vi "copyScriptToTestDir.vi"(8 "error in (no error)":errorcluster, 10 "Path in":path, 11 "FileNeologist in":refnum<class "FileNeologist.lvclass">) -> (0 "error out":errorcluster, 2 "Path out":path, 3 "FileNeologist out":refnum<class "FileNeologist.lvclass">)   [LabVIEW 2011, in "Tools.lvlib" / "Filing.lvlib" / "FileNeologist.lvclass"]
uses:
  FileNeologist.lvclass
  FileNeologist.lvclass/FileNeologist.ctl
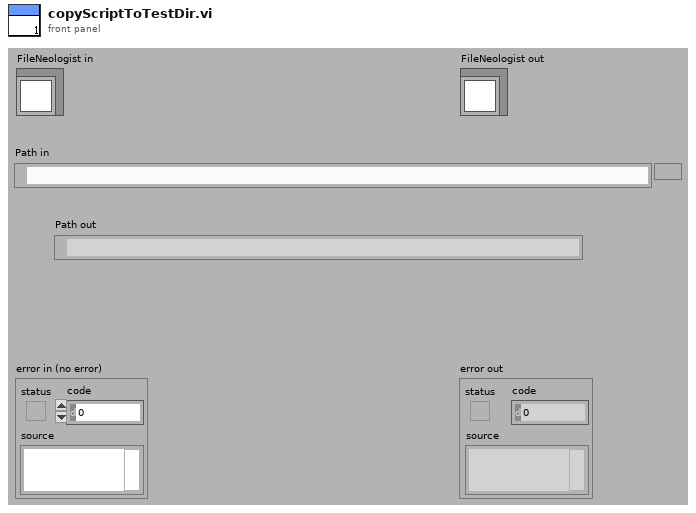
[diagram p1: front panel]
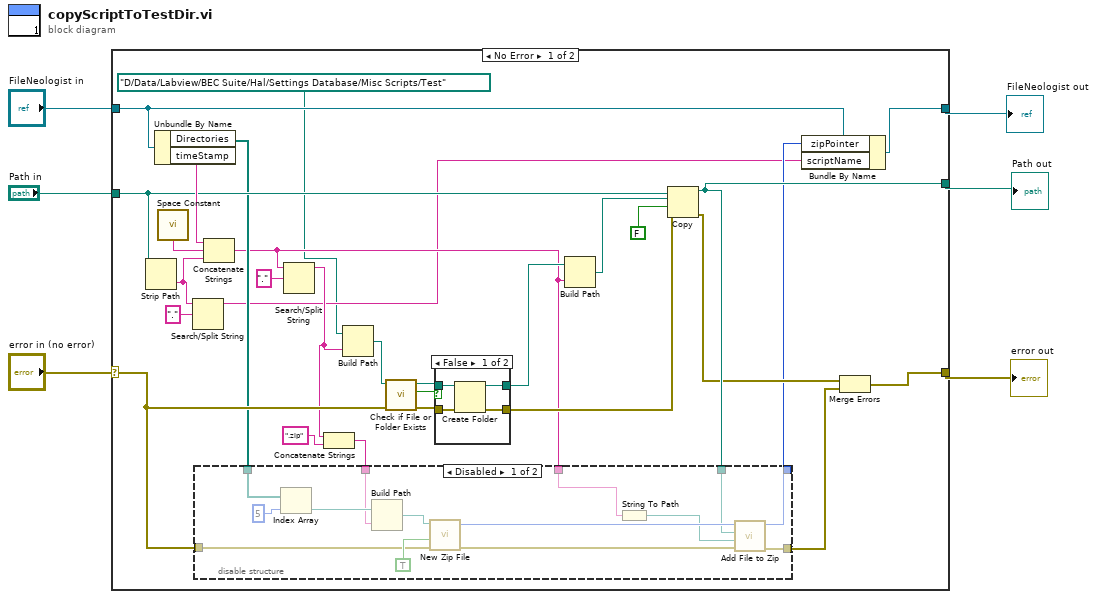
[diagram p0: block diagram]
diagram:
  n1 = case shown="No Error" "error in (no error)" {
    selector: "error in (no error)" -> [w23 w57]
    tunnel: [w20 w57] -> w5
    tunnel: [w11 w56] -> w3
    tunnel: "FileNeologist in" -> [w12 w56]
    tunnel: "Path in" -> [w25 _]
    tunnel: [w22 _] -> w1
    frame No Error {
      n2 = Strip Path(path=w25) -> (name=w9:string)  [unwired: 1 out]
      n3 = Unbundle By Name(w12) -> ("Directories"=w21:path[], "timeStamp"=w26:string)
      n4 = call <vilib>:"Space Constant.vi"() -> ("String"=w34:string)
      n5 = Search/Split String(string=w9, search string/char (-)=".") -> (substring before match=w8:string)  [unwired: 1 in, 2 out]
      n6 = Concatenate Strings(w26, w34, w9) -> (w18:string)
      n7 = Search/Split String(string=w18, search string/char (-)=".") -> (substring before match=w17:string)  [unwired: 1 in, 2 out]
      n8 = Concatenate Strings(w17, ".zip") -> (w15:string)
      n9 = Build Path(base path=path "D:/Data/Labview/BEC Suite/Hal/Settings Database/Misc Scripts/Test", name or relative path=w17) -> (appended path=w29:path)
      n10 = call <vilib>:"Check if File or Folder Exists.vi"("error in (no error)"=w23, "path"=w29) -> ("error out"=w30:errorcluster, "file or folder exists?"=w32:bool, "dup path"=w31:path)  [unwired: 7 in]
      n11 = case shown="False" w32 {
        tunnel: w31 -> [w53 w55]
        tunnel: [w50 w55] -> w28
        tunnel: w30 -> [w52 w54]
        tunnel: [w51 w54] -> w27
        frame False {
          n12 = Create Folder(path (use dialog)=w53, error in=w52) -> (created path=w50:path, error out=w51:errorcluster)  [unwired: 1 in, 1 out]
        }
        frame True {
        }
      }
      n13 = Build Path(base path=w28, name or relative path=w18) -> (appended path=w33:path)
      n14 = Copy(8:w27, 9:FALSE, 10:w33, 11:w25) -> (0:w19:errorcluster, 3:w22:path)  [unwired: 1 in, 1 out]
      n15 = disable-structure shown="Disabled" {
        disable-tunnel: w23 -> [w48 _]
        disable-tunnel: w22 -> [w46 _]
        disable-tunnel: w21 -> [w45 _]
        disable-tunnel: w18 -> [w39 _]
        disable-tunnel: w15 -> [w38 _]
        disable-tunnel: [w37 _] -> w14
        disable-tunnel: [w36 _] -> w13
        frame Disabled {
          n16 = Index Array(array=w45, index=5) -> (element=w43:path)
          n17 = Build Path(base path=w43, name or relative path=w38) -> (appended path=w42:path)
          n18 = call <vilib>:"New Zip File.vi"("error in (no error)"=w48, "confirm overwrite? (F)"=TRUE, "target"=w42) -> ("error out"=w41:errorcluster, "zip file out"=w47:i64)  [unwired: 2 in, 1 out]
          n19 = String To Path(string=w39) -> (path=w40:path)
          n20 = call <vilib>:"Add File to Zip.vi"("error in (no error)"=w41, "destination path in zip"=w40, "source file path"=w46, "zip file in"=w47) -> ("error out"=w37:errorcluster, "zip file out"=w36:i64)  [unwired: 6 in]
        }
        frame Enabled {
        }
      }
      n21 = Bundle By Name(cluster=w12, "zipPointer"=w13, "scriptName"=w8) -> (w11:refnum<class "FileNeologist.lvclass">)
      n22 = Merge Errors(w19, w14) -> (w20:errorcluster)
    }
    frame Error {
    }
  }
  "error out" <- w5
  "FileNeologist out" <- w3
  "Path out" <- w1
